vi "AMX-画矩形.vi"(7 "布尔":bool, 8 "error in (no error)":errorcluster caption="错误输入（无错误）", 10 "颗粒物位置坐标":cluster{"X":dbl, "Y":dbl}[](array[cluster]) {"Y" format="%.2f"; "X" format="%.2f"}, 11 "Image In":T1(plugin-control)) -> (0 "error out":errorcluster caption="错误输出", 3 "Image Out":T1(plugin-control))   [LabVIEW 2017]
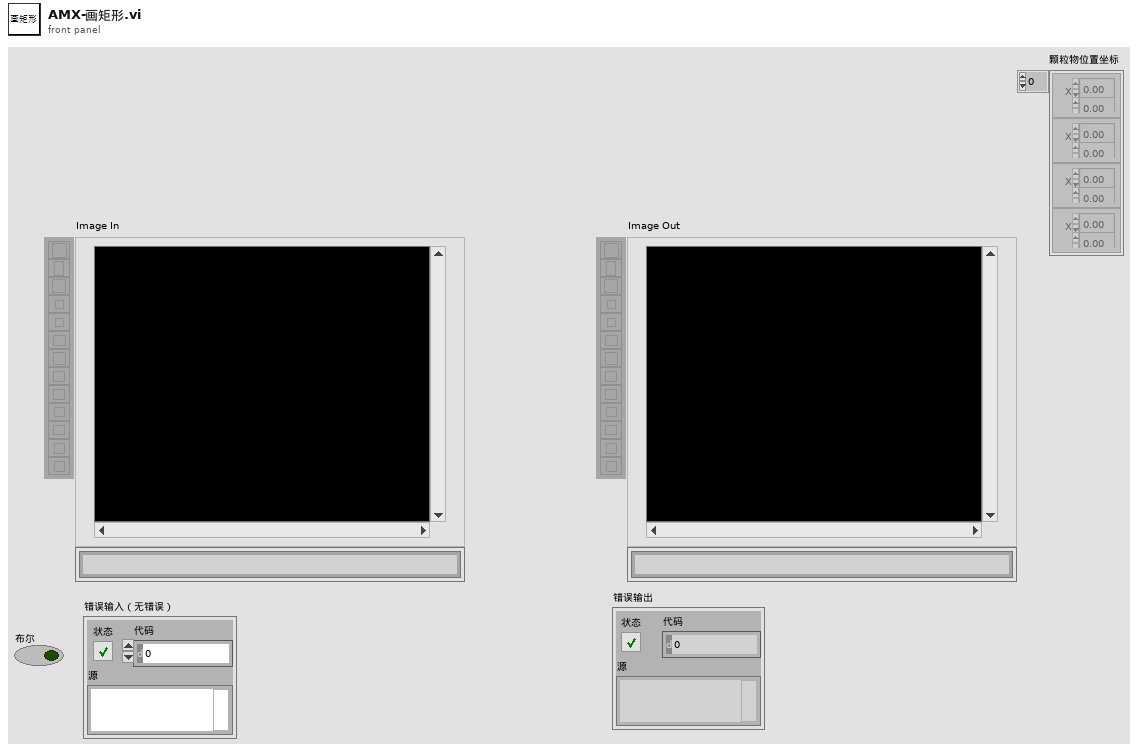
[diagram p1: front panel]
types:
  T1 = typedef "IMAQ Image.ctl" = refnum<image>
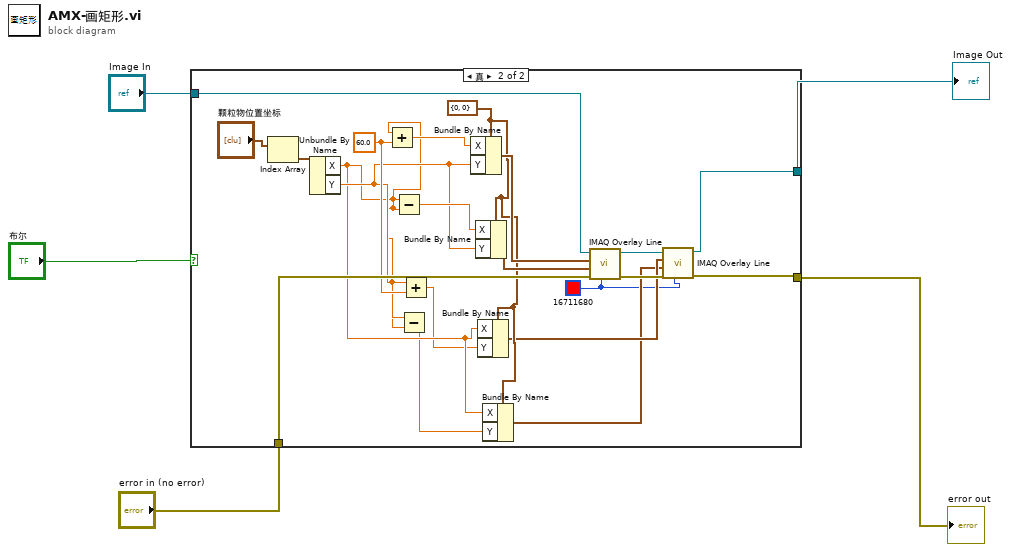
[diagram p0: block diagram]
diagram:
  n1 = case shown="真" "布尔" {
    tunnel: "Image In" -> [w7 w28]
    tunnel: [w7 w24] -> w4
    tunnel: "error in (no error)" -> [w6 w27]
    tunnel: [w6 w23] -> w2
    frame False {
    }
    frame True {
      w8 = u32 16711680 ("Color")
      w14 = cluster{"X":i32, "Y":i32} {"X"=0, "Y"=0} ("Start Point")
      w20 = 60.0 ("y")
      n2 = Index Array(array="颗粒物位置坐标") -> (element=w21:cluster{"X":dbl, "Y":dbl})  [unwired: 1 in]
      n3 = Unbundle By Name(w21) -> ("X"=w13:dbl, "Y"=w15:dbl)
      n4 = Add(x=w13, y=w20) -> (x+y=w19:dbl)
      n5 = Subtract(x=w13, y=w13) -> (x-y=w17:dbl)
      n6 = Subtract(x=w15, y=w13) -> (x-y=w11:dbl)
      n7 = Add(x=w15, y=w20) -> (x+y=w12:dbl)
      n8 = Bundle By Name(cluster=w14, "X"=w19, "Y"=w15) -> (w18:cluster{"X":i32, "Y":i32})
      n9 = Bundle By Name(cluster=w14, "X"=w17, "Y"=w15) -> (w16:cluster{"X":i32, "Y":i32})
      n10 = Bundle By Name(cluster=w14, "X"=w13, "Y"=w12) -> (w10:cluster{"X":i32, "Y":i32})
      n11 = Bundle By Name(cluster=w14, "X"=w13, "Y"=w11) -> (w9:cluster{"X":i32, "Y":i32})
      n12 = call "IMAQ Overlay Line"("Color"=w8, "error in (no error)"=w27, "End Point"=w16, "Start Point"=w18, "Image"=w28) -> ("error out"=w25:errorcluster, "Image Out"=w26:T1)  [unwired: 5 in]
      n13 = call "IMAQ Overlay Line"("Color"=w8, "error in (no error)"=w25, "End Point"=w9, "Start Point"=w10, "Image"=w26) -> ("error out"=w23:errorcluster, "Image Out"=w24:T1)  [unwired: 5 in]
    }
  }
  "Image Out" <- w4
  "error out" <- w2
